vi "test_UDP Protocol Factory.vi"(8 "error in (no error)":errorcluster, 11 "TestCase in":refnum<class "Instrument Addon Scripting API Protocol Factories Unit Tests.lvclass">) -> (0 "error out":errorcluster, 3 "TestCase out":refnum<class "Instrument Addon Scripting API Protocol Factories Unit Tests.lvclass">)   [LabVIEW 2023, in "Instrument Addon Scripting API Protocol Factories Unit Tests.lvclass"]
uses:
  Instrument Addon Scripting API Protocol Factories Unit Tests.lvclass
  <vilib>/addons/_JKI Toolkits/VI Tester/TestCase.llb/TestCase.lvclass
  UDP/UDP.lvclass
  UDP/UDP Settings.ctl
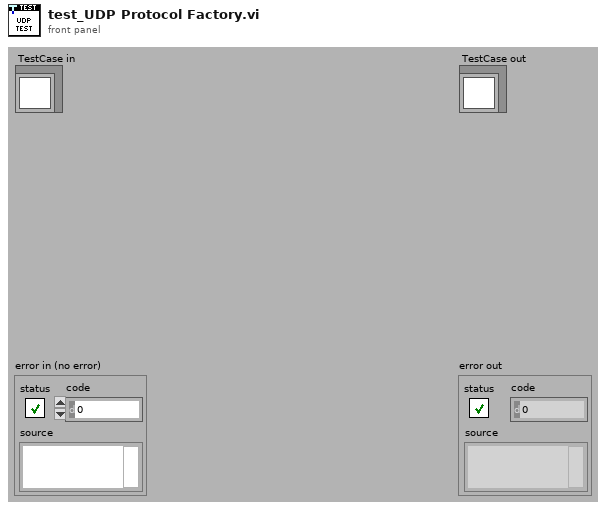
[diagram p1: front panel]
types:
  T1 = typedef "Protocols.lvlib/UDP.lvclass/UDP Settings.ctl" = cluster{"Local IP Address":string, "Local Port":u16, "Target IP Address":string, "Target Port":u16}
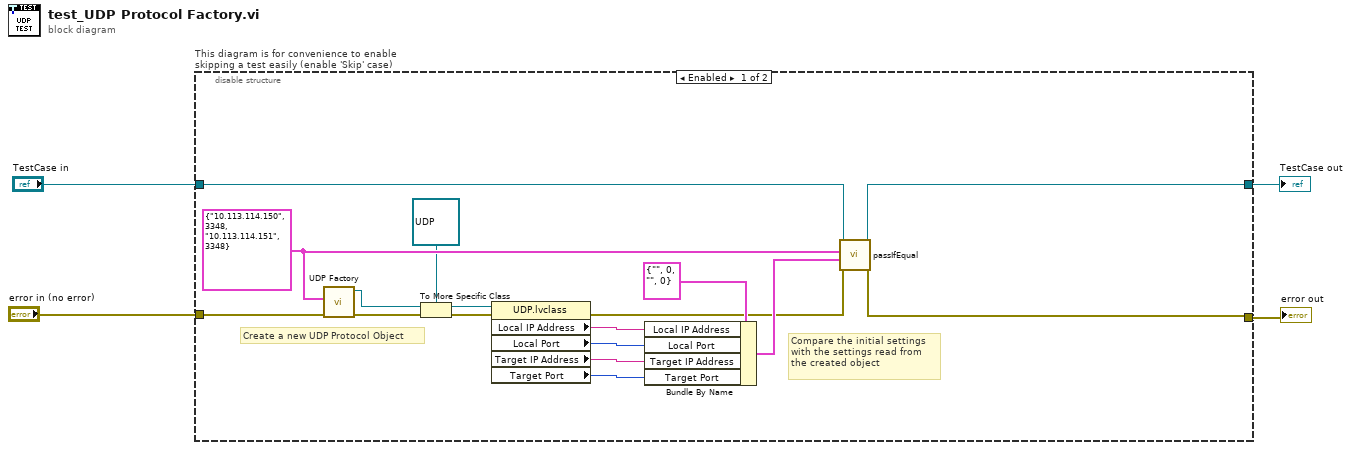
[diagram p0: block diagram]
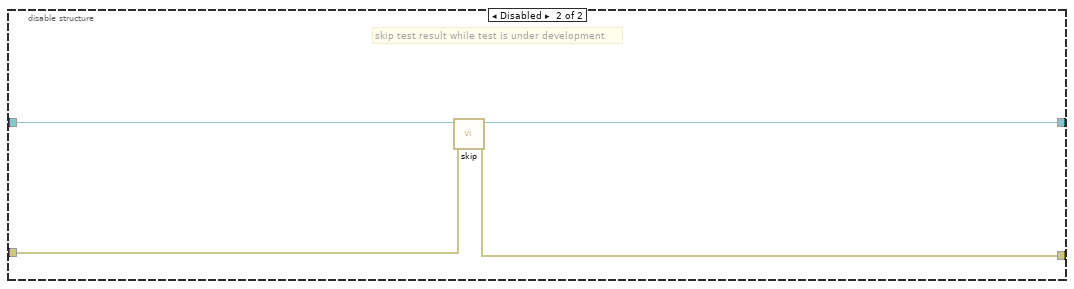
[diagram p2: hidden frame]
diagram:
  n1 = disable-structure "This diagram is for convenience to enable skipping a test easily (enable 'Skip' case)" shown="Enabled" {
    disable-tunnel: "TestCase in" -> [w21 w25]
    disable-tunnel: [w20 w23] -> w1
    disable-tunnel: [w19 w24] -> w3
    disable-tunnel: "error in (no error)" -> [w18 w22]
    frame Enabled {
      w17 = T1 {"Local IP Address"="10.113.114.150", "Local Port"=3348, "Target IP Address"="10.113.114.151", "Target Port"=3348} ("UPD Settings")
      # "Compare the initial settings \nwith the settings read from \nthe created object"
      # "Create a new UDP Protocol Object"
      n2 = call "UDP Factory.vi"("error in (no error)"=w18, "UDP settings"=w17) -> ("error out"=w7:errorcluster, "protocol out"=w6:refnum<class "Protocol Parent.lvclass">)  [unwired: 8 in]
      n3 = To More Specific Class(target class=refnum<class "UDP.lvclass"> refnum ("Protocols.lvlib:UDP.lvclass"), reference=w6, error in=w7) -> (specific class reference=w9:refnum<class "UDP.lvclass">, error out=w8:errorcluster)
      n4 = property class="UDP.lvclass"(reference=w9, error in=w8) -> (error out=w14:errorcluster, "Local IP Address"=w13:string, "Local Port"=w12:u16, "Target IP Address"=w11:string, "Target Port"=w10:u16)  [unwired: 1 out]
      n5 = Bundle By Name(cluster=T1 {"Local IP Address"="", "Local Port"=0, "Target IP Address"="", "Target Port"=0} ("UPD Settings"), "Local IP Address"=w13, "Local Port"=w12, "Target IP Address"=w11, "Target Port"=w10) -> (w15:T1)
      n6 = call-dynamic "passIfEqual.vi"("error in (no error)"=w14, "y"=w15, "x"=w17, "TestCase in"=w21) -> ("error out"=w19:errorcluster, "TestCase out"=w20:refnum<class "Instrument Addon Scripting API Protocol Factories Unit Tests.lvclass">)  [unwired: 6 in]
    }
    frame Disabled {
      # "skip test result while test is under development"
      n7 = call <vilib>:"skip.vi"("error in (no error)"=w22, "TestCase in"=w25) -> ("error out"=w24:errorcluster, "TestCase out"=w23:refnum<class "Instrument Addon Scripting API Protocol Factories Unit Tests.lvclass">)  [unwired: 8 in]
    }
  }
  "error out" <- w3
  "TestCase out" <- w1
